vi "SetScale.vi"(1 "# A/D bits":i16, 2 "Display mode":T1=enum."Log Grey Scale") -> (0 "Array":cluster{dbl, u32}[](array[cluster]))   [LabVIEW 2022 SP3]
uses:
  ScaleMethod.ctl
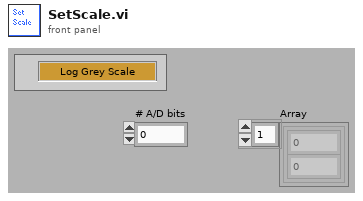
[diagram p1: front panel]
types:
  T1 = typedef "ScaleMethod.ctl" = enum16{"Linear Abs Grey", "Log Grey Scale", "Linear Color Scale", "dB Scale", "Verasonics Doppler"}
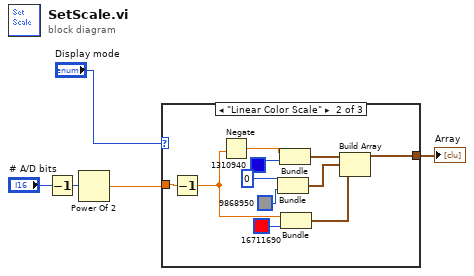
[diagram p0: block diagram]
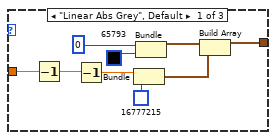
[diagram p2: hidden frame]
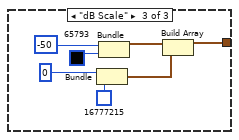
[diagram p3: hidden frame]
diagram:
  n1 = Decrement(x="# A/D bits") -> (x-1=w3:i16)
  n2 = Power Of 2(x=w3) -> (2^x=w5:dbl)
  n3 = case shown="\"Linear Color Scale\"" "Display mode" {
    tunnel: [w8 w17 w27] -> w2
    tunnel: w5 -> [w7 w16 _]
    frame "Linear Abs Grey", Default {
      n4 = Decrement(x=w7) -> (x-1=w6:dbl)
      n5 = Decrement(x=w6) -> (x-1=w11:dbl)
      n6 = Bundle(w11, u32 16777215) -> (w9:cluster{dbl, u32})  [unwired: 1 out]
      n7 = Bundle(0, u32 65793) -> (w10:cluster{i32, u32})  [unwired: 1 out]
      n8 = Build Array(w10, w9) -> (w8:cluster{dbl, u32}[])
    }
    frame "Linear Color Scale" {
      n9 = Decrement(x=w16) -> (x-1=w15:dbl)
      n10 = Negate(x=w15) -> (-x=w21:dbl)
      n11 = Bundle(0, u32 9868950) -> (w19:cluster{i32, u32})  [unwired: 1 out]
      n12 = Bundle(w21, u32 1310940) -> (w20:cluster{dbl, u32})  [unwired: 1 out]
      n13 = Bundle(w15, u32 16711690) -> (w18:cluster{dbl, u32})  [unwired: 1 out]
      n14 = Build Array(w20, w19, w18) -> (w17:cluster{dbl, u32}[])
    }
    frame "dB Scale" {
      n15 = Bundle(0, u32 16777215) -> (w28:cluster{i32, u32})  [unwired: 1 out]
      n16 = Bundle(-50, u32 65793) -> (w29:cluster{i32, u32})  [unwired: 1 out]
      n17 = Build Array(w29, w28) -> (w27:cluster{i32, u32}[])
    }
  }
  "Array" <- w2
